vi "InitHH_UIThread.vi"(8 "error in (no error)":errorcluster, 9 "mode":T2 items=["Histo"=0, "T2"=2, "T3"=3, "Conti"=8], 10 "refsource":T3, 11 "Library Version":string="3.0") -> (0 "error out":errorcluster, 2 "Init Info":T1, 3 "DevIdx":i32)   [LabVIEW 2017]
uses:
  HH_RefSource.ctl
  HH_MeasMode.ctl
  HH_InitInfo.ctl
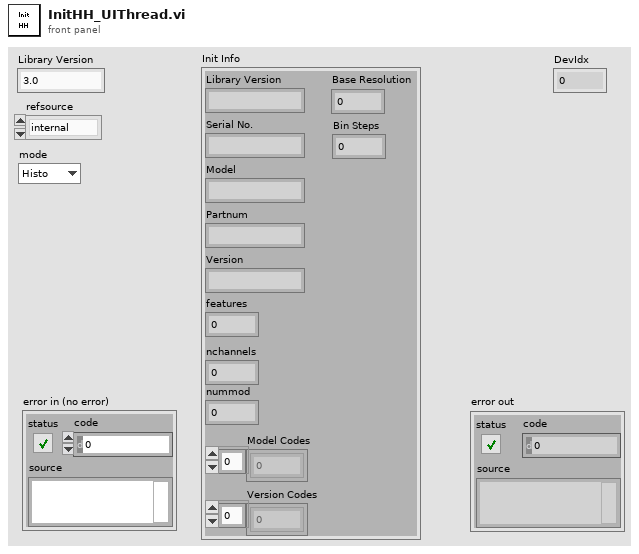
[diagram p1: front panel]
types:
  T1 = typedef "HH_InitInfo.ctl" = cluster{"Library Version":string, "Serial No.":string, "Model":string, "Partnum":string, "Version":string, "features":i32, "nchannels":i32, "nummod":i32, "Model Codes":i32[], "Version Codes":i32[], "Base Resolution":dbl, "Bin Steps":i32}
  T2 = typedef "HH_MeasMode.ctl" = i32
  T3 = typedef "HH_RefSource.ctl" = enum16{"internal", "external"}
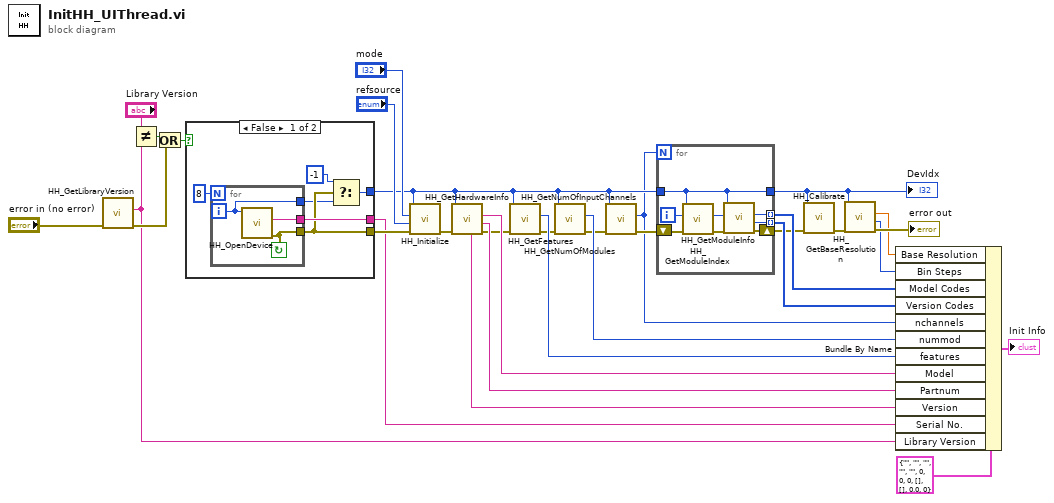
[diagram p0: block diagram]
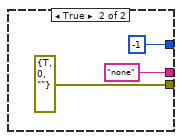
[diagram p2: hidden frame]
diagram:
  n1 = call "HH_GetLibraryVersion.vi"("error in (no error)"="error in (no error)") -> ("error out"=w31:errorcluster, "Version"=w18:string)  [unwired: 8 in, 1 out]
  n2 = Not Equal?(x="Library Version", y=w18) -> (x != y?=w30:bool)
  n3 = Or(x=w30, y=w31) -> (x .or. y?=w29:bool)
  n4 = case shown="False" w29 {
    tunnel: [w34 -1 ("return type")] -> w11
    tunnel: [w37 "none" ("serial")] -> w20
    tunnel: [w36 errorcluster {"status"=TRUE, "code"=0, "source"=""} ("error out")] -> w28
    frame False {
      n5 = for {
        N: 8 -> [_]
        tunnel: [w40] -> w36
        tunnel: [w39] -> w37
        tunnel: [w41] -> w35
        i -> [w41]
        stop <- w40 continue-if-true
        n6 = call "HH_OpenDevice.vi"("devidx"=w41) -> ("error out"=w40:errorcluster, "serial"=w39:string)  [unwired: 8 in, 1 out]
      }
      n7 = Select(t=-1, s=w36, f=w35) -> (s? t:f=w34:i32)
    }
    frame True {
    }
  }
  n8 = call "HH_Initialize.vi"("error in (no error)"=w28, "refsource"="refsource", "mode"="mode", "devidx"=w11) -> ("error out"=w25:errorcluster)  [unwired: 6 in, 1 out]
  n9 = call "HH_GetHardwareInfo.vi"("error in (no error)"=w25, "devidx"=w11) -> ("error out"=w16:errorcluster, "Partnum"=w23:string, "Model"=w24:string, "Version"=w22:string)  [unwired: 5 in, 1 out]
  n10 = call "HH_GetFeatures.vi"("error in (no error)"=w16, "devidx"=w11) -> ("error out"=w15:errorcluster, "features"=w21:i32)  [unwired: 7 in, 1 out]
  n11 = call "HH_GetNumOfModules.vi"("error in (no error)"=w15, "devidx"=w11) -> ("error out"=w13:errorcluster, "nummod"=w14:i32)  [unwired: 7 in, 1 out]
  n12 = call "HH_GetNumOfInputChannels.vi"("error in (no error)"=w13, "devidx"=w11) -> ("error out"=w12:errorcluster, "nchannels"=w10:i32)  [unwired: 7 in, 1 out]
  n13 = for {
    N: w10 -> [_]
    tunnel: w11 -> [w46]
    tunnel: [w49] -> w9 mode=indexing
    tunnel: [w48] -> w8 mode=indexing
    tunnel: [w46] -> w5
    shift-right: [w45] -> w7
    shift-left: w12 -> [w52]
    i -> [w47]
    n14 = call "HH_GetModuleIndex.vi"("error in (no error)"=w52, "channel"=w47, "devidx"=w46) -> ("error out"=w50:errorcluster, "modidx"=w51:i32)  [unwired: 6 in, 1 out]
    n15 = call "HH_GetModuleInfo.vi"("error in (no error)"=w50, "modidx"=w51, "devidx"=w46) -> ("error out"=w45:errorcluster, "versioncode"=w49:i32, "modelcode"=w48:i32)  [unwired: 5 in, 1 out]
  }
  "DevIdx" <- w5
  n16 = call "HH_Calibrate.vi"("error in (no error)"=w7, "devidx"=w5) -> ("error out"=w6:errorcluster)  [unwired: 8 in, 1 out]
  n17 = call "HH_GetBaseResolution.vi"("error in (no error)"=w6, "devidx"=w5) -> ("error out"=→"error out":errorcluster, "binsteps"=w3:i32, "resolution"=w2:dbl)  [unwired: 6 in, 1 out]
  n18 = Bundle By Name(cluster=T1 {"Library Version"="", "Serial No."="", "Model"="", "Partnum"="", "Version"="", "features"=0, "nchannels"=0, "nummod"=0, "Model Codes"=[], "Version Codes"=[], "Base Resolution"=0.0, "Bin Steps"=0} ("Init"), "Base Resolution"=w2, "Bin Steps"=w3, "Model Codes"=w8, "Version Codes"=w9, "nchannels"=w10, "nummod"=w14, "features"=w21, "Model"=w24, "Partnum"=w23, "Version"=w22, "Serial No."=w20, "Library Version"=w18) -> (→"Init Info":T1)
